vi "Open LabVIEW File.vi"(8 "error in":errorcluster, 11 "File Info in":T1) -> (0 "error out":errorcluster, 3 "File Info out":T1)   [LabVIEW 2020, in "Peer Review.lvclass"]
uses:
  Peer Review.lvclass
  TypeDefs/File Info.ctl
  TypeDefs/File State.ctl
  TypeDefs/VI Type.ctl
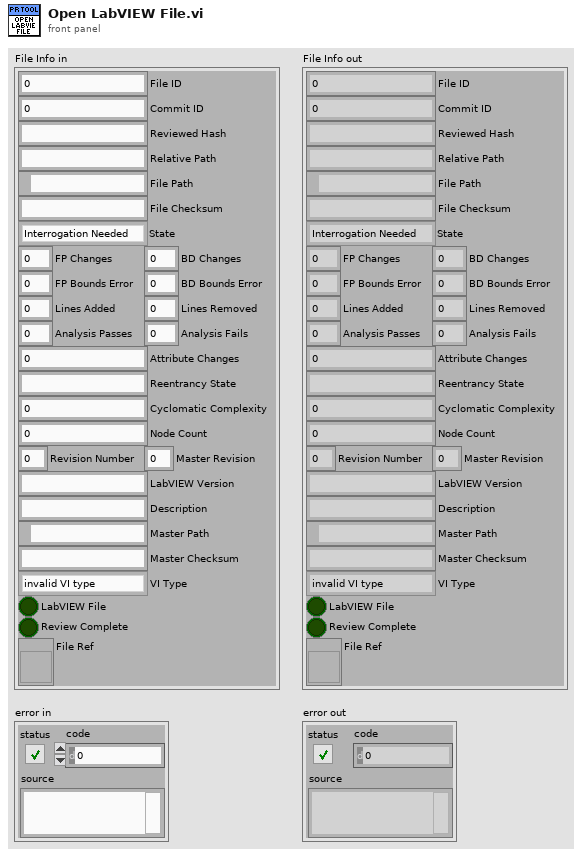
[diagram p1: front panel]
types:
  T1 = typedef "Peer Review.lvclass/File Info.ctl" = cluster{"File ID":i32, "Commit ID":i32, "Reviewed Hash":string, "Relative Path":string, "File Path":path, "File Checksum":string, "State":T2, "FP Changes":i32, "BD Changes":i32, "FP Bounds Error":dbl, "BD Bounds Error":dbl, "Lines Added":i32, "Lines Removed":i32, "Analysis Passes":i32, "Analysis Fails":i32, "Attribute Changes":i32, "Reentrancy State":string, "Cyclomatic Complexity":i32, "Node Count":i32, "Revision Number":u32, "LabVIEW Version":string, "Description":string, "Master Path":path, "Master Checksum":string, "VI Type":T3, "LabVIEW File":bool, "Review Complete":bool, "File Ref":refnum<vi>, "Master Revision":u32}
  T2 = typedef "Peer Review.lvclass/File State.ctl" = enum16{"Interrogation Needed", "Modified", "Deleted", "Added", "Matches Previous", "No Changes", "Moved", "Empty File"}
  T3 = typedef "Peer Review.lvclass/VI Type.ctl" = enum32{"invalid VI type", "Standard VI", "Control VI", "Global VI", "Polymorphic VI", "Configuration VI", "SubSystem", "Facade VI", "Method VI", "Statechart Diagram VI"}
  T4 = enum32{"invalid VI type", "Standard VI", "Control VI", "Global VI", "Polymorphic VI", "Configuration VI", "SubSystem", "Facade VI", "Method VI", "Statechart Diagram VI"}
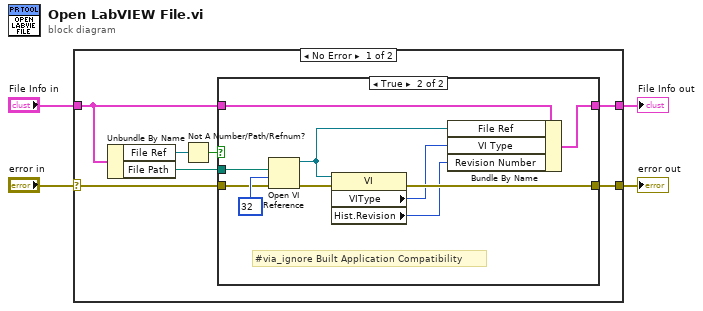
[diagram p0: block diagram]
diagram:
  n1 = case shown="No Error" "error in" {
    selector: "error in" -> [w9 w25]
    tunnel: [w11 w24] -> w4
    tunnel: [w10 w25] -> w3
    tunnel: "File Info in" -> [w8 w24]
    frame No Error {
      n2 = Unbundle By Name(w8) -> ("File Ref"=w6:refnum<vi>, "File Path"=w7:path)
      n3 = Not A Number/Path/Refnum?(number/path/refnum=w6) -> (NaN/Path/Refnum?=w5:bool)
      n4 = case shown="True" w5 {
        tunnel: [w12 w23] -> w11
        tunnel: [w13 w22] -> w10
        tunnel: w9 -> [w13 w17]
        tunnel: w8 -> [w12 w16]
        tunnel: w7 -> [_ w15]
        frame False {
          # "File is already opened, so do nothing."
        }
        frame True {
          # "#via_ignore Built Application Compatibility"
          n5 = Open VI Reference(vi path=w15, options=32, error in (no error)=w17) -> (vi reference=w19:refnum<vi>, error out=w21:errorcluster)  [unwired: 1 in, 2 out]
          n6 = property on="Property Node" class="VI"(reference=w19, error in=w21) -> (error out=w22:errorcluster, "VIType"=w20:T4, "Hist.Revision"=w14:u32)  [unwired: 1 out]
          n7 = Bundle By Name(cluster=w16, "File Ref"=w19, "VI Type"=w20, "Revision Number"=w14) -> (w23:T1)
        }
      }
    }
    frame Error {
    }
  }
  "File Info out" <- w4
  "error out" <- w3
